vi "Log.vi"(8 "error in (no error)":errorcluster, 9 "message":string, 11 "WebSocket Connection in":refnum<class "WebSocket Connection.lvclass">) -> (0 "error out":errorcluster, 3 "WebSocket Connection out":refnum<class "WebSocket Connection.lvclass">)   [LabVIEW 2019, in "WebSocket Server Toolkit.lvlib" / "WebSocket Connection.lvclass"]
doc: "<b>Description</b> Log a message to the server log.\n\n<b>Inputs</b>\n<b>message</b>: Message to send to the server log. A timestamp and connection information will be prepended to the messsage."
uses:
  WebSocket Connection.lvclass
  WebSocket Connection.lvclass/WebSocket Connection.ctl
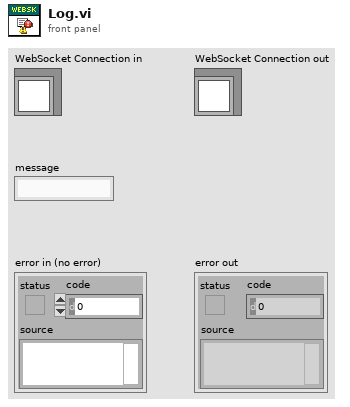
[diagram p1: front panel]
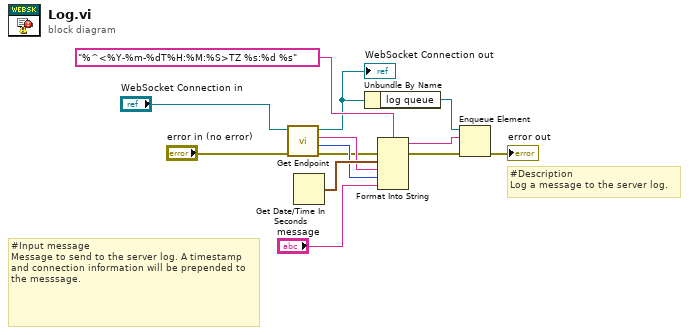
[diagram p0: block diagram]
diagram:
  # "#Input message\nMessage to send to the server log. A timestamp and connection information will be prepended to the messsage."
  # "#Description\nLog a message to the server log."
  n1 = call "Get Endpoint.vi"("error in (no error)"="error in (no error)", "WebSocket Connection in"="WebSocket Connection in") -> ("error out"=w7:errorcluster, "remote port"=w8:u16, "remote address"=w9:string, "WebSocket Connection out"=w5:refnum<class "WebSocket Connection.lvclass">)  [unwired: 6 in]
  "WebSocket Connection out" <- w5
  n2 = Get Date/Time In Seconds() -> (seconds since 1Jan1904=w12:timestamp)
  n3 = Unbundle By Name(w5) -> ("log queue"=w4:refnum<queue>)
  n4 = Format Into String(format string="%^<%Y-%m-%dT%H:%M:%S>TZ %s:%d %s", error in=w7, w12, w9, w8, "message") -> (resulting string=w3:string, error out=w2:errorcluster)  [unwired: 1 in]
  n5 = Enqueue Element(queue=w4, element=w3, error in (no error)=w2) -> (error out=→"error out":errorcluster)  [unwired: 1 in, 2 out]
